vi "New_Magazine_Globals.vi"() -> ()   [LabVIEW 2019]
uses:
  New_Magazine_Cluster.ctl
  New_Magazine_Control_States.ctl
  <vilib>/Rock Robotics/WPI/Solenoid/WPI_SolenoidValue.ctl
  Utility_VIs/Basic_Motor_Modes.ctl
panel:
  in  "New_Magazine_Motor_Mode":T1
  in  "New_Magazine_Pneumatic":T2
  in  "New_Magazine_Motor_Power":dbl
  in  "New_Magazine_Spun_Up":refnum<notifier>
  in  "New_Magazine_Set_Notifier":refnum<notifier>
  in  "New_Magazine_Execute_Notifier":refnum<notifier>
  in  "New_Magazine_Execute_Ref":string="New_Magazine_Execute_Ref"
  in  "New_Magazine_Set_Ref":string="New_Magazine_Set_Ref"
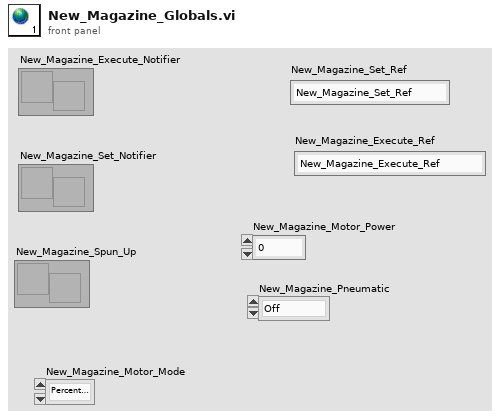
[diagram p1: front panel]
types:
  T1 = typedef "Basic_Motor_Modes.ctl" = enum16{"Percent_Voltage", "Speed_Control", "Position_Control", "Current"}
  T2 = typedef "WPI_SolenoidValue.ctl" = enum16{"Off", "On", "Forward", "Reverse"}
diagram:
